vi "HoldEM.vi"(10 "Requested EM":bool) -> (2 "EM out":bool)   [LabVIEW 2017]
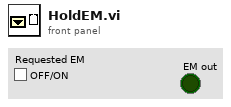
[diagram p1: front panel]
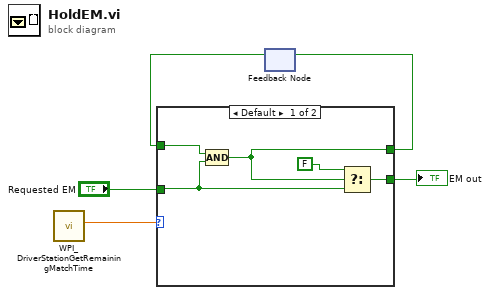
[diagram p0: block diagram]
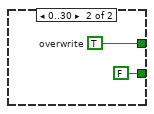
[diagram p2: hidden frame]
diagram:
  n1 = call <vilib>:"WPI_DriverStationGetRemainingMatchTime.vi"() -> ("Match Time(s)"=w1:sgl)  [unwired: 10 in, 1 out]
  n2 = feedback #1() -> (w2:bool)  [unwired: 1 in]
  n3 = case shown="Default" w1 {
    tunnel: [w10 FALSE ("Requested EM")] -> w4
    tunnel: "Requested EM" -> [w6 _]
    tunnel: w2 -> [w8 _]
    tunnel: [w7 w12] -> w3
    frame Default {
      n4 = Compound Arithmetic op=AND(w8, w6) -> (w7:bool)
      n5 = Select(t=FALSE, s=w7, f=w6) -> (s? t:f=w10:bool)
    }
    frame 0..30 {
      w12 = TRUE  # overwrite
    }
  }
  "EM out" <- w4
  n6 = feedback-in #1(w3) -> ()
